vi "Read.vi"(8 "Error In":errorcluster, 10 "DI Channel":u8, 11 "LINX Resource":T1) -> (0 "Error Out":errorcluster, 1 "Centimeters":dbl, 2 "Inches":dbl, 3 "LINX Resource":T1)   [LabVIEW 2011, in "LVH-LINX.lvlib" / "GH-311.lvlib"]
uses:
  GH-311.lvlib
  Private/Type Defs/LINX Ref.ctl
  Private/Type Defs/Platform.ctl
  Private/Type Defs/Interface.ctl
  Private/Device/Type Defs/LINX Device Config.ctl
  Private/Device/Type Defs/TCP Config.ctl
  Private/Type Defs/Device Family.ctl
  LVH-LINX.lvlib
  Private/Device/Device.lvlib
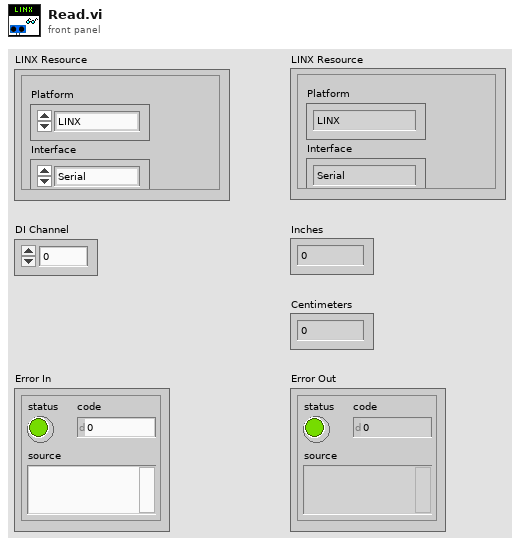
[diagram p1: front panel]
types:
  T1 = typedef "LVH-LINX.lvlib/LINX Ref.ctl" = cluster{"Platform":T2, "Interface":T3, "LINX Device Config":T4}
  T2 = typedef "LVH-LINX.lvlib/Platform.ctl" = enum16{"LINX", "myRIO"}
  T3 = typedef "LVH-LINX.lvlib/Interface.ctl" = enum16{"Serial", "TCP"}
  T4 = typedef "LVH-LINX.lvlib/Device.lvlib/LINX Device Config.ctl" = cluster{"Interface":T3, "COM Port":refnum<visa-resource-name>, "TCP Configuration":T5, "Device Family":T6, "Device ID":u8, "Device Name":string, "TCP Ref":refnum<k5>}
  T5 = typedef "LVH-LINX.lvlib/Device.lvlib/TCP Config.ctl" = cluster{"IP Address":string, "Port":u16}
  T6 = typedef "LVH-LINX.lvlib/Device Family.ctl" = enum8{"National Instruments", "Digilent", "Arduino"}
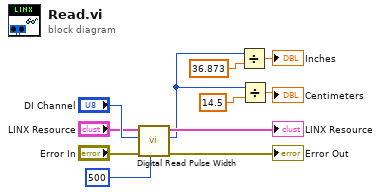
[diagram p0: block diagram]
diagram:
  n1 = call "Digital Read Pulse Width.vi"("Timeout  (250 mS)"=u32 500, "Error In"="Error In", "DI Channel"="DI Channel", "LINX Resource"="LINX Resource") -> ("Error Out"=→"Error Out":errorcluster, "Pulse Width (uS)"=w2:u32, "LINX Resource"=→"LINX Resource":T1)  [unwired: 5 in]
  n2 = Divide(x=w2, y=36.873) -> (x/y=→"Inches":dbl)
  n3 = Divide(x=w2, y=14.5) -> (x/y=→"Centimeters":dbl)
